vi "Update Value.vi"(6 "Time":dbl, 8 "error in (no error)":errorcluster, 11 "2WayValve in":refnum<class "2WayValveV.lvclass">) -> (0 "error out":errorcluster, 1 "Update":bool, 2 "Value":variant, 3 "2WayValve out":refnum<class "2WayValveV.lvclass">)   [LabVIEW 2020, in "VolatusGUIElements.lvlib" / "2WayValveV.lvclass"]
uses:
  2WayValveV.lvclass
  2WayValveV.lvclass/2WayValveV.ctl
  Command Picture.vi
  Feedback Picture.vi
  Energized Picture.vi
  Picture.vi
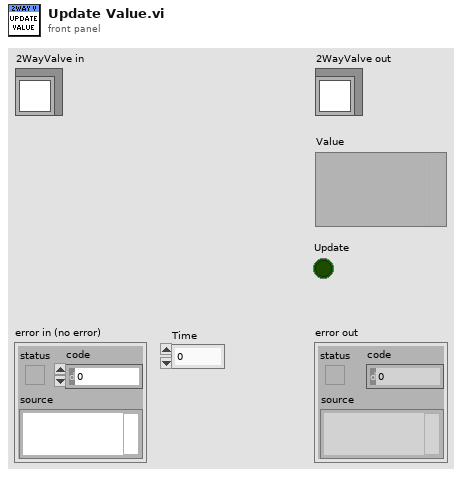
[diagram p1: front panel]
types:
  T1 = typedef "VolatusGUIElements.lvlib/2WayValveV.lvclass/Values.ctl" = cluster{"Command":T2, "CmdFB":T2, "Closed":T2, "Open":T2, "Energized":T2}
  T2 = typedef "VolatusGUIElements.lvlib/2WayValveV.lvclass/Channel State.ctl" = cluster{"Value":bool, "Stale":bool, "Config":bool, "Error":bool, "Prev":bool}
  T3 = typedef "VolatusGUIElements.lvlib/2WayValveV.lvclass/Unused Element.ctl" = cluster{"Command":bool, "Feedback":bool, "Energized":bool}
  T4 = typedef "VolatusGUIElements.lvlib/2WayValveV.lvclass/Picture.ctl" = enum16{"Blank", "OutClose", "OutOpen", "OutTranClose", "OutTranOpen", "OutConfig", "OutStale", "OutError", "InClose", "InOpen", "InTranClose", "InTranOpen", "InConfig", "InStale", "InError", "EnOff", "EnOn", "EnConfig", "EnStale", "EnError"}
  T5 = typedef "VolatusGUIElements.lvlib/2WayValveV.lvclass/Valve Pictures.ctl" = cluster{"Command":T6, "Feedback":T7, "Energized":T8}
  T6 = typedef "VolatusGUIElements.lvlib/2WayValveV.lvclass/Command Pictures.ctl" = cluster{"Error":T4, "Config":T4, "Stale":T4, "Close":T4, "Open":T4, "TranClose":T4, "TranOpen":T4}
  T7 = typedef "VolatusGUIElements.lvlib/2WayValveV.lvclass/Feedback Pictures.ctl" = cluster{"Error":T4, "Config":T4, "Stale":T4, "Closed":T4, "Open":T4, "TranClose":T4, "TranOpen":T4}
  T8 = typedef "VolatusGUIElements.lvlib/2WayValveV.lvclass/Energized Pictures.ctl" = cluster{"Error":T4, "Config":T4, "Stale":T4, "False":T4, "True":T4}
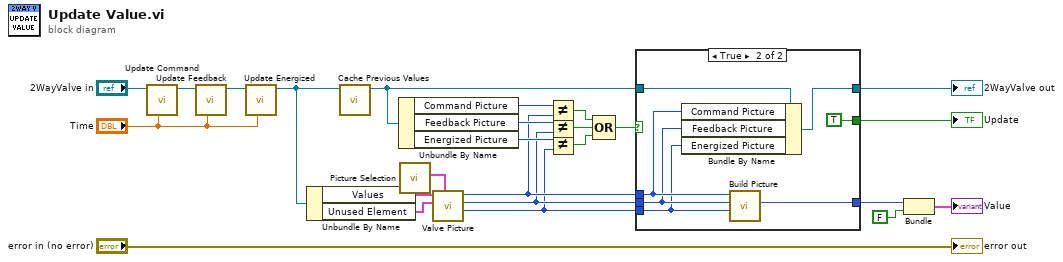
[diagram p0: block diagram]
diagram:
  n1 = call "Update Command.vi"("Time"="Time", "2WayValve in"="2WayValve in") -> ("2WayValve out"=w23:refnum<class "2WayValveV.lvclass">)  [unwired: 8 in, 1 out]
  n2 = call "Update Feedback.vi"("Time"="Time", "2WayValve in"=w23) -> ("2WayValve out"=w22:refnum<class "2WayValveV.lvclass">)  [unwired: 8 in, 1 out]
  n3 = call "Update Energized.vi"("Time"="Time", "2WayValve in"=w22) -> ("2WayValve out"=w20:refnum<class "2WayValveV.lvclass">)  [unwired: 8 in, 1 out]
  n4 = Unbundle By Name(w20) -> ("Values"=w17:T1, "Unused Element"=w19:T3)
  n5 = call "Cache Previous Values.vi"("2WayValve in"=w20) -> ("2WayValve out"=w8:refnum<class "2WayValveV.lvclass">)  [unwired: 9 in, 1 out]
  n6 = Unbundle By Name(w8) -> ("Command Picture"=w14:T4, "Feedback Picture"=w13:T4, "Energized Picture"=w12:T4)
  n7 = call "Picture Selection.vi"() -> ("Valve Pictures"=w18:T5)  [unwired: 11 in]
  n8 = call "Valve Picture.vi"("Valve Pictures"=w18, "Unused Element"=w19, "Values"=w17) -> ("Energized Picture"=w2:T4, "Feedback Picture"=w3:T4, "Command Picture"=w4:T4)  [unwired: 6 in]
  n9 = Not Equal?(x=w14, y=w4) -> (x != y?=w9:bool)
  n10 = Not Equal?(x=w13, y=w3) -> (x != y?=w11:bool)
  n11 = Not Equal?(x=w12, y=w2) -> (x != y?=w10:bool)
  n12 = Compound Arithmetic op=OR(w9, w11, w10) -> (w7:bool)
  n13 = case shown="True" w7 {
    tunnel: w8 -> [w26 w31]
    tunnel: [_ TRUE] -> w6
    tunnel: [_ w32] -> w5
    tunnel: w4 -> [_ w30]
    tunnel: w3 -> [_ w29]
    tunnel: w2 -> [_ w28]
    tunnel: [w26 w27] -> w1
    frame False {
    }
    frame True {
      n14 = Bundle By Name(cluster=w31, "Command Picture"=w30, "Feedback Picture"=w29, "Energized Picture"=w28) -> (w27:refnum<class "2WayValveV.lvclass">)
      n15 = call "Build Picture.vi"("Energized Picture"=w28, "Feedback Picture"=w29, "Command Picture"=w30) -> ("Valve Picture"=w32:picture)  [unwired: 8 in]
    }
  }
  "2WayValve out" <- w1
  "Update" <- w6
  n16 = Bundle("Valve Picture"=w5, FALSE) -> (→"Value":cluster{"Valve Picture":picture, bool})  [unwired: 1 in]
  "error out" <- "error in (no error)"
